vi "write_to_text_file.vi"(7 "delimiter (\\t)":string="\t", 8 "error in (no error)":errorcluster, 10 "file (use dialog)":path, 11 "PointCollection in":refnum<class "PointCollection.lvclass">) -> (0 "error out":errorcluster, 3 "PointCollection out":refnum<class "PointCollection.lvclass">)   [LabVIEW 2010, in "PointCollection.lvclass"]
uses:
  PointCollection.lvclass
  mode_enum.ctl
  <vilib>/Utility/file.llb/Write To Spreadsheet File (DBL).vi
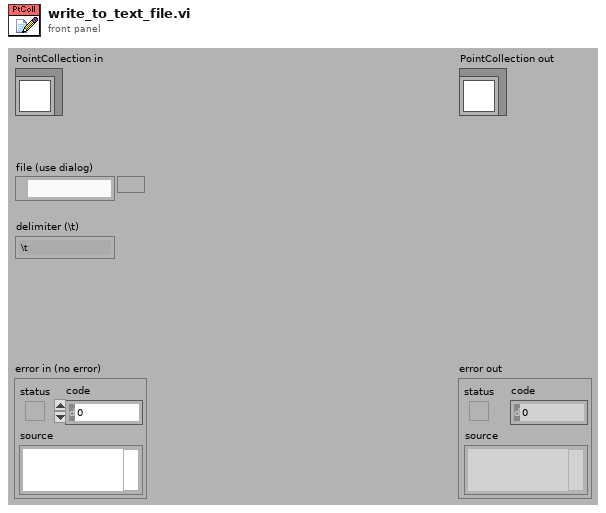
[diagram p1: front panel]
types:
  T1 = typedef "PointCollection.lvclass/mode_enum.ctl" = enum16{"points first", "dimensions first"}
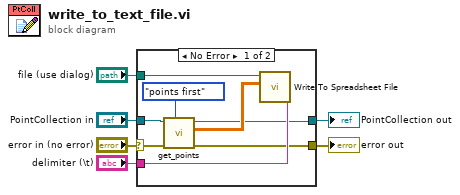
[diagram p0: block diagram]
diagram:
  n1 = case shown="No Error" "error in (no error)" {
    selector: "error in (no error)" -> [w12 w16]
    tunnel: [w9 w16] -> w5
    tunnel: [w8 w15] -> w3
    tunnel: "PointCollection in" -> [w11 w15]
    tunnel: "file (use dialog)" -> [w14 _]
    tunnel: "delimiter (\\t)" -> [w13 _]
    frame No Error {
      n2 = call-dynamic "get_points.vi"("retrieval mode"=mode_enum."points first", "error in (no error)"=w12, "PointCollection in"=w11) -> ("error out"=w9:errorcluster, "points"=w10:dbl[][], "PointCollection out"=w8:refnum<class "PointCollection.lvclass">)  [unwired: 6 in]
      n3 = call-poly <vilib>:"Write To Spreadsheet File.vi"("delimiter (\\t)"=w13, "2D data"=w10, "file path (dialog if empty)"=w14) -> ()  [unwired: 5 in, 1 out]
    }
    frame Error {
    }
  }
  "error out" <- w5
  "PointCollection out" <- w3
